vi "FolderMon update.vi"(4 "error in (no error)":errorcluster, 5 "FolderMonitoring":T1[](array[typedef]), 6 "Polling (-1:  Unchanged)":i32=-1, 7 "daemon VI Ref":refnum<vi>) -> (0 "error out":errorcluster, 3 "dup daemon VI Ref":refnum<vi>)   [LabVIEW 2011]
uses:
  FolderMon config.ctl
  FolderMon events.ctl
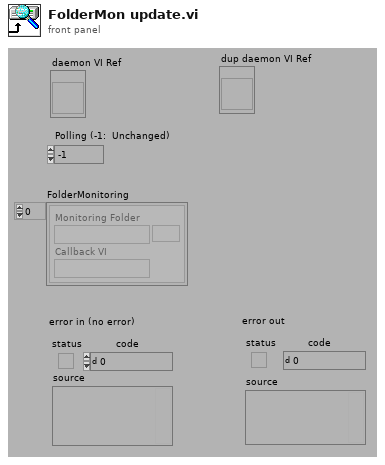
[diagram p1: front panel]
types:
  T1 = typedef "FolderMon config.ctl" = cluster{"Monitoring Folder":path, "Callback VI":string}
  T2 = typedef "FolderMon events.ctl" = enum16{"stop", "update"}
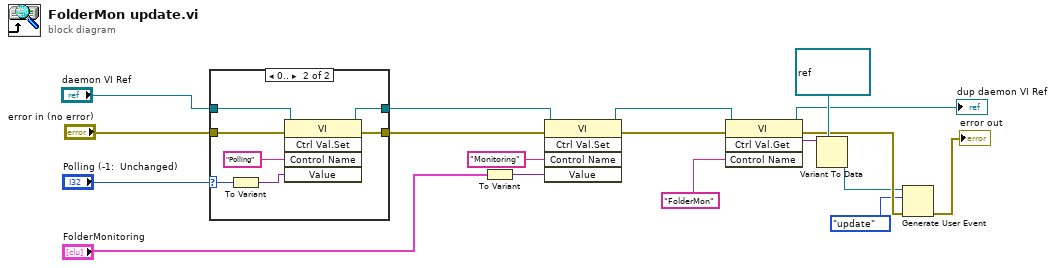
[diagram p0: block diagram]
diagram:
  w16 = refnum<user-event> refnum items=["stop", "update"] ("FolderMon")
  n1 = case shown="0.." "Polling (-1:  Unchanged)" {
    selector: "Polling (-1:  Unchanged)" -> [_ w21]
    tunnel: "error in (no error)" -> [w20 w26]
    tunnel: [w20 w25] -> w9
    tunnel: "daemon VI Ref" -> [w19 w23]
    tunnel: [w19 w22] -> w8
    frame -1, Default {
    }
    frame 0.. {
      n2 = To Variant(anything=w21) -> (Variant=w24:variant)
      n3 = invoke class="VI" method="Ctrl Val.Set"(reference=w23, error in=w26, "Control Name"="Polling", "Value"=w24) -> (reference out=w22:refnum<vi>, error out=w25:errorcluster)  [unwired: 1 in, 3 out]
    }
  }
  n4 = To Variant(anything="FolderMonitoring") -> (Variant=w1:variant)
  n5 = invoke class="VI" method="Ctrl Val.Set"(reference=w8, error in=w9, "Control Name"="Monitoring", "Value"=w1) -> (reference out=w7:refnum<vi>, error out=w10:errorcluster)  [unwired: 1 in, 3 out]
  n6 = invoke class="VI" method="Ctrl Val.Get"(reference=w7, error in=w10, "Control Name"="FolderMon") -> (reference out=→"dup daemon VI Ref":refnum<vi>, error out=w15:errorcluster, "Get Control Value Variant"=w17:variant)  [unwired: 1 in, 1 out]
  n7 = Variant To Data(type=w16, Variant=w17) -> (data=w14:refnum<user-event>)  [unwired: 1 in, 1 out]
  n8 = Generate User Event(user event=w14, event data cluster=FolderMon_events."update" ("event data"), error in=w15) -> (error out=→"error out":errorcluster)  [unwired: 1 out]
